vi "SUB_COM1_CTRLC.vi"(3 "VISA resource name":refnum<visa-resource-name>) -> (0 "error out":errorcluster, 1 "duplicate VISA resource name":refnum<visa-resource-name>)   [LabVIEW 2011]
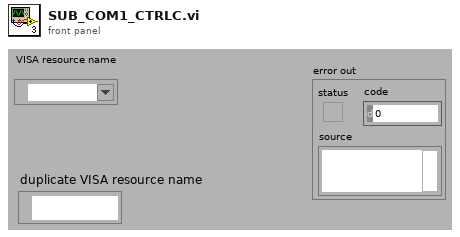
[diagram p1: front panel]
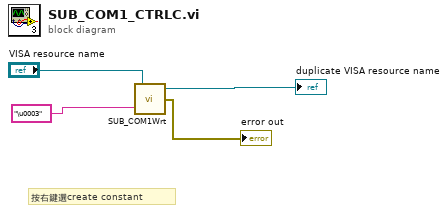
[diagram p0: block diagram]
diagram:
  # "按右鍵選create constant"
  n1 = call "SUB_COM1Wrt.vi"("VISA resource name"="VISA resource name", "write buffer"="\u0003") -> ("duplicate VISA resource name"=→"duplicate VISA resource name":refnum<visa-resource-name>, "error out"=→"error out":errorcluster)  [unwired: 1 out]
